vi "set controls.vi"() -> ()   [LabVIEW 2019]
uses:
  Controller/F.L.Y Stick Controller Global.vi
  Drive Global.vi
panel:
  in  "X":dbl=1.0
  in  "Z":dbl=1.0
  in  "y":dbl=1.0
  in  "Drive Command":T1
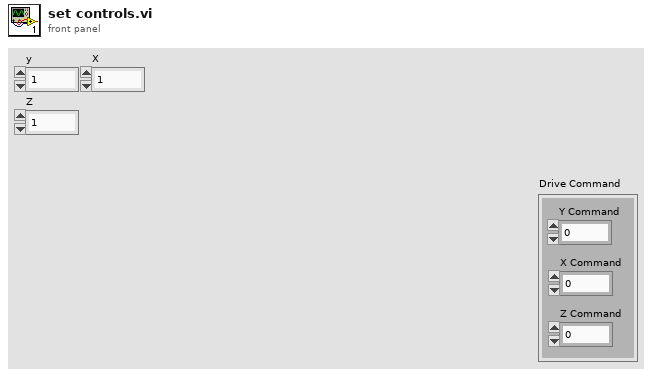
[diagram p1: front panel]
types:
  T1 = cluster{"Y Command":dbl, "X Command":dbl, "Z Command":dbl}
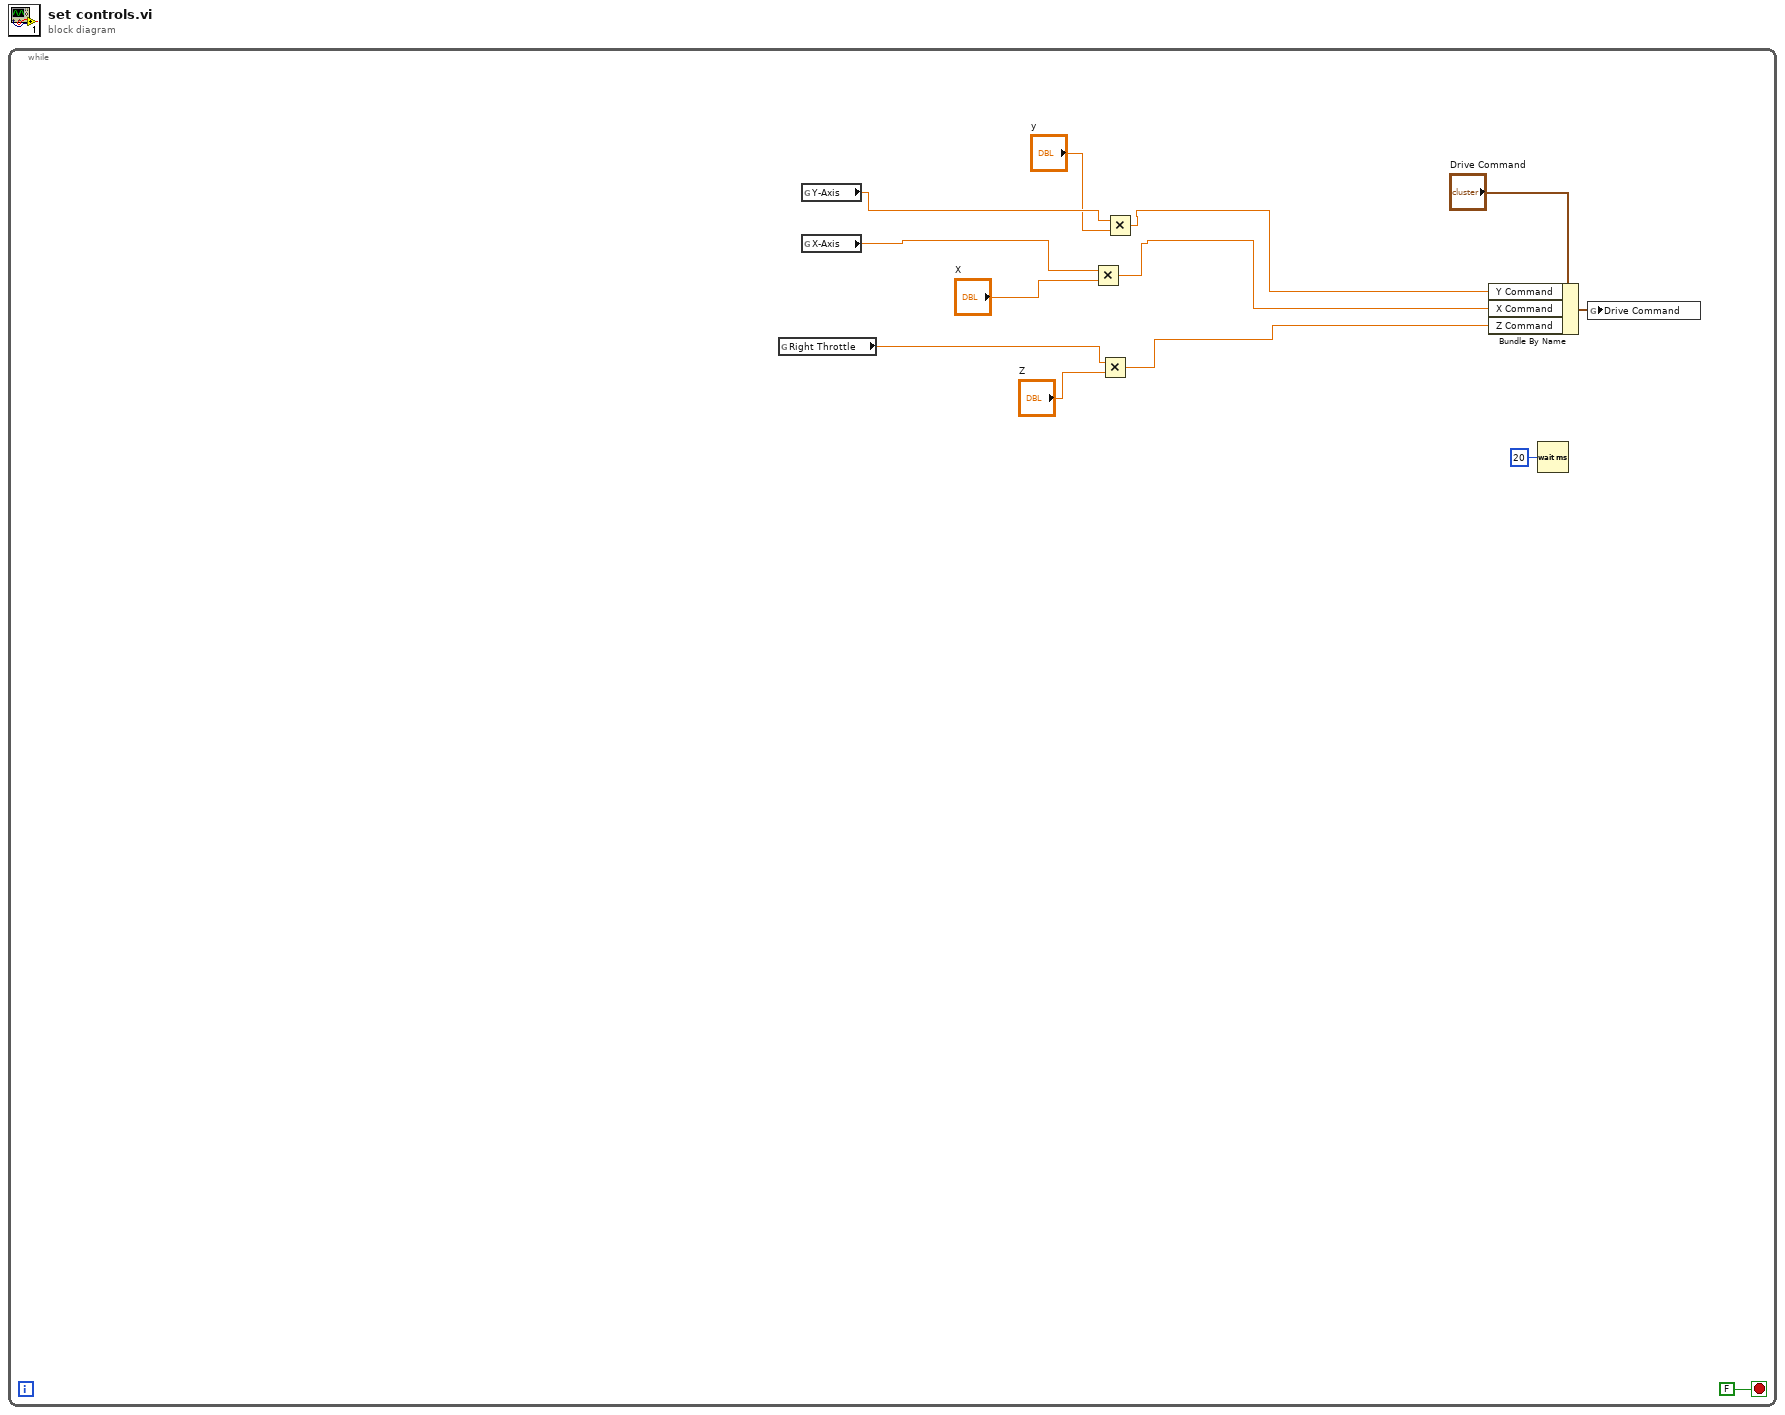
[diagram p0: block diagram]
diagram:
  n1 = while {
    stop <- FALSE stop-if-true
    n2 = global read "F.L.Y Stick Controller Global.vi" "Right Throttle"() -> (w5:dbl)
    n3 = global read "F.L.Y Stick Controller Global.vi" "Y-Axis"() -> (w9:dbl)
    n4 = global read "F.L.Y Stick Controller Global.vi" "X-Axis"() -> (w3:dbl)
    n5 = Multiply(x=w3, y="X") -> (x*y=w2:dbl)
    n6 = Multiply(x=w5, y="Z") -> (x*y=w6:dbl)
    n7 = Multiply(x=w9, y="y") -> (x*y=w8:dbl)
    n8 = Bundle By Name(cluster="Drive Command", "Y Command"=w8, "X Command"=w2, "Z Command"=w6) -> (w11:T1)
    n9 = Wait (ms)(milliseconds to wait=u32 20) -> ()  [unwired: 1 out]
    n10 = global write "Drive Global.vi" "Drive Command"(w11) -> ()
  }
